vi "Get Most Recent Frame (if active).vi"(8 "error in (no error)":errorcluster, 11 "Orca-Flash 4.0 V2 in":refnum<class "Orca-Flash 4.0 V2.lvclass">) -> (0 "error out":errorcluster, 3 "Orca-Flash 4.0 V2 out":refnum<class "Orca-Flash 4.0 V2.lvclass">)   [LabVIEW 2018, in "Orca-Flash 4.0 V2.lvlib" / "Orca-Flash 4.0 V2.lvclass"]
uses:
  Orca-Flash 4.0 V2.lvclass
  C:/LVCUR/flash-gordon/Hardware/Camera/Camera.lvclass
  Orca-Flash 4.0 V2.lvclass/Orca-Flash 4.0 V2.ctl
  Resources/GLOBAL/GLOBAL Time-critical.vi
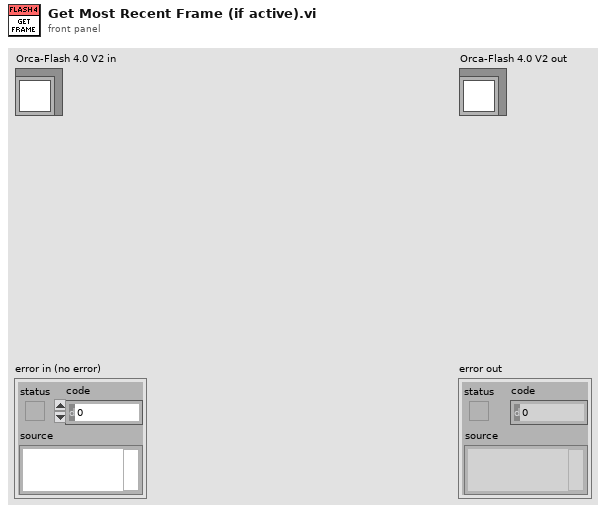
[diagram p1: front panel]
types:
  T1 = typedef "Physical Camera Assignment.ctl" = cluster{"Channel Name":string, "Camera Type":T2, "Serial Number":string, "Flip Vertically":bool, "Flip Horizontally":bool, "photonsPerCount":dbl, "wavelength":i16}
  T2 = typedef "Camera Type.ctl" = enum16{"Orca-Flash 4.0 V2"}
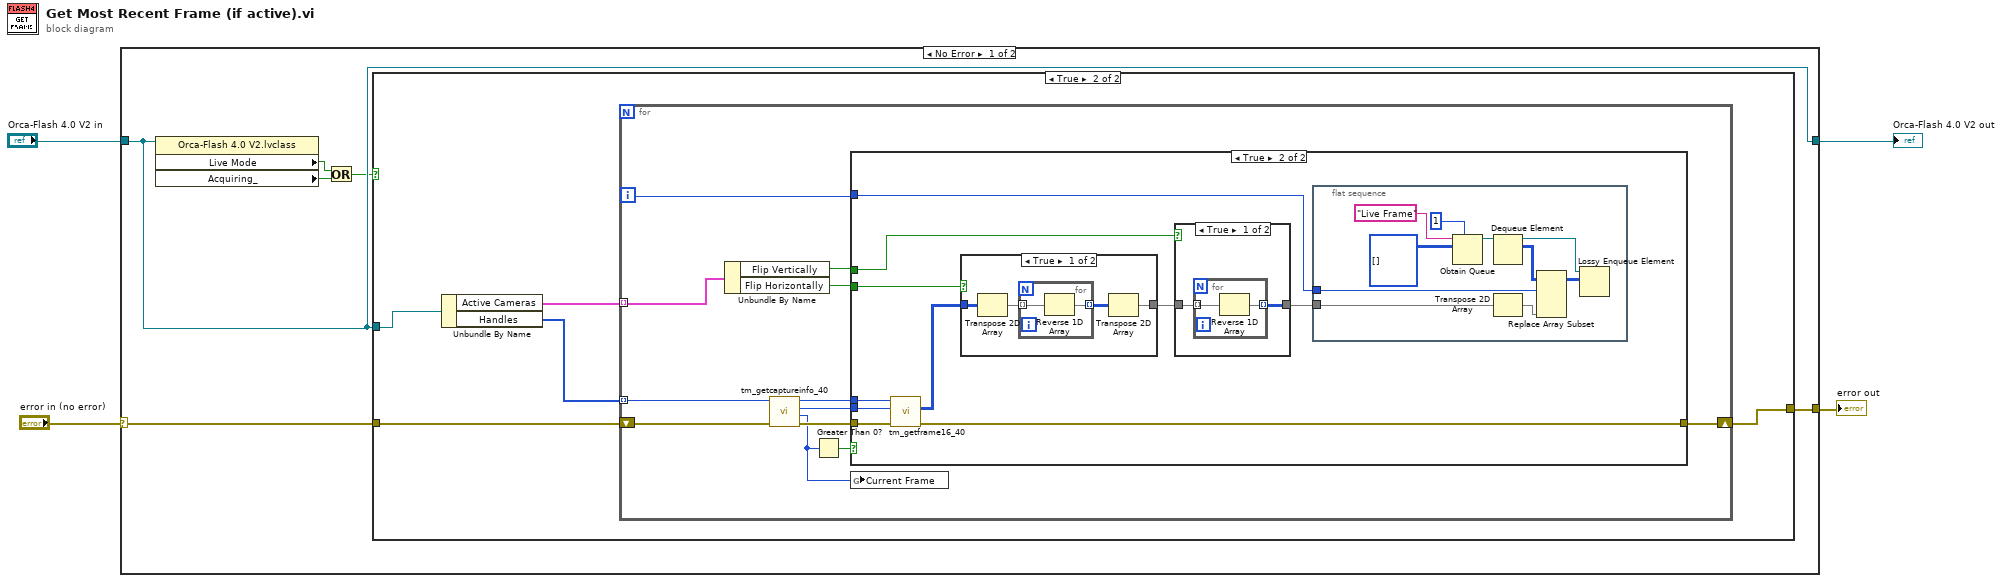
[diagram p0: block diagram]
diagram:
  n1 = case shown="No Error" "error in (no error)" {
    selector: "error in (no error)" -> [w8 w63]
    tunnel: [w7 w63] -> w3
    tunnel: [w9 w62] -> w1
    tunnel: "Orca-Flash 4.0 V2 in" -> [w9 w62]
    frame No Error {
      n2 = property class="Orca-Flash 4.0 V2.lvclass"(reference=w9) -> ("Live Mode"=w10:bool, "Acquiring_"=w5:bool)  [unwired: 1 in, 2 out]
      n3 = Or(x=w10, y=w5) -> (x .or. y?=w6:bool)
      n4 = case shown="True" w6 {
        tunnel: w9 -> [_ w16]
        tunnel: w8 -> [w11 w14]
        tunnel: [w11 w15] -> w7
        frame False {
        }
        frame True {
          n5 = Unbundle By Name(w16) -> ("Active Cameras"=w12:T1[], "Handles"=w13:u32[])
          n6 = for {
            tunnel: w13 -> [w21] mode=indexing
            shift-right: [w28] -> w15
            shift-left: w14 -> [w22]
            tunnel: w12 -> [w17] mode=indexing
            i -> [w18]
            n7 = Unbundle By Name(w17) -> ("Flip Vertically"=w20:bool, "Flip Horizontally"=w19:bool)
            n8 = call <userlib>:"tm_getcaptureinfo_40.vi"("error in (no error)"=w22, "Handle in"=w21) -> ("error out"=w26:errorcluster, "Frame Count"=w23:i32, "Frame Index"=w24:i32, "Handle out"=w25:u32)  [unwired: 6 in]
            n9 = Greater Than 0?(x=w23) -> (x > 0?=w27:bool)
            n10 = case shown="True" w27 {
              tunnel: [w29 w30] -> w28
              tunnel: w18 -> [_ w39]
              tunnel: w20 -> [_ w36]
              tunnel: w19 -> [_ w35]
              tunnel: w26 -> [w29 w34]
              tunnel: w25 -> [_ w33]
              tunnel: w24 -> [_ w32]
              frame False {
              }
              frame True {
                n11 = call <userlib>:"tm_getframe16_40.vi"("error in (no error)"=w34, "Frame Index"=w32, "Handle in"=w33) -> ("error out"=w30:errorcluster, "Data"=w31:u16[][])  [unwired: 5 in, 2 out]
                n12 = case shown="True" w35 {
                  tunnel: w31 -> [w57 w61]
                  tunnel: [w55 w61] -> w38
                  frame True {
                    n13 = Transpose 2D Array(2D array=w57) -> (transposed array=w58:u16[][])
                    n14 = for {
                      tunnel: w58 -> [w60] mode=indexing
                      tunnel: [w59] -> w56 mode=indexing
                      n15 = Reverse 1D Array(array=w60) -> (reversed array=w59:u16[])
                    }
                    n16 = Transpose 2D Array(2D array=w56) -> (transposed array=w55:u16[][])
                  }
                  frame False {
                  }
                }
                n17 = case shown="True" w36 {
                  tunnel: w38 -> [w50 w54]
                  tunnel: [w51 w54] -> w37
                  frame True {
                    n18 = for {
                      tunnel: w50 -> [w53] mode=indexing
                      tunnel: [w52] -> w51 mode=indexing
                      n19 = Reverse 1D Array(array=w53) -> (reversed array=w52:u16[])
                    }
                  }
                  frame False {
                  }
                }
                n20 = flat-sequence {
                  tunnel: w39 -> [w49]
                  tunnel: w37 -> [w48]
                  frame #0 {
                    n21 = Obtain Queue(max queue size (-1, unlimited)=1, name (unnamed)="Live Frame", element data type=u16[][][] [] ("output array")) -> (queue out=w43:refnum<queue>)  [unwired: 2 in, 2 out]
                    n22 = Dequeue Element(queue=w43) -> (queue out=w40:refnum<queue>, element=w41:u16[][][])  [unwired: 2 in, 2 out]
                    n23 = Transpose 2D Array(2D array=w48) -> (transposed array=w47:u16[][])
                    n24 = Replace Array Subset(array=w41, new element=w47, index (dim 0)=w49) -> (w44:u16[][][])  [unwired: 2 in]
                    n25 = Lossy Enqueue Element(queue=w40, element=w44) -> ()  [unwired: 1 in, 4 out]
                  }
                }
              }
            }
            n26 = global write "GLOBAL Time-critical.vi" "Current Frame"(w23) -> ()
          }
        }
      }
    }
    frame Error {
    }
  }
  "error out" <- w3
  "Orca-Flash 4.0 V2 out" <- w1
